vi "Programmablauf.vi"(8 "error in (no error)":errorcluster caption="Fehler (Eingang, kein Fehler)", 11 "AK Trigger":bool) -> (0 "error out":errorcluster caption="Fehler (Ausgang)")   [LabVIEW 2020, in "Schedule Modul.lvlib"]
uses:
  Schedule Modul.lvlib
  Aktion Trigger Freigabe.ctl
  Aktion FGV Testdaten sammeln.ctl
  T90/Aktion FGV Automatic Start.ctl
  Sprachverwaltung/FGV Aktion Tabelle zerlegen.ctl
  Aktion FGV Scheduler Status.ctl
  Aktion FGV Schedule Daten.ctl
  Funktionstasten/Funktionstasten-Aktion.ctl
  Funktionstasten/Zustaende.ctl
  Aktion FGV Schedule Log.ctl
  Auto Kalibrieren/VI Auto Kalibrieren.vi
  Seiten/Erweiterte Konfig/Dichtheitstest.vi
  Seiten/Erweiterte Konfig/Konfig CG-Check/CG-Test.vi
  T90/T90 main.vi
  Funktionstasten/Funktionstasten.lvlib
  Funktionstasten/Freigabe Aktionen.ctl
  AK-Schnittstelle/AK-Schnittstelle.lvlib
  Allgemein/allgemeine Sub-VIs.lvlib
  Seiten/Erweiterte Konfig/Erweiterte Konfig.lvlib
  Seiten/Erweiterte Konfig/Konfig CG-Check/CG-Check Konfig.lvlib
  T90/T90.lvlib
  Sprachverwaltung/Sprachverwaltung.lvlib
  Auto Kalibrieren/Auto Kalibrieren.lvlib
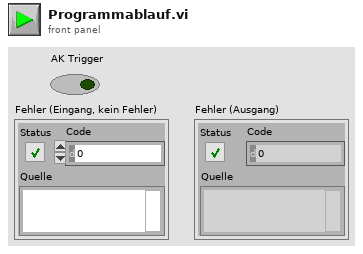
[diagram p1: front panel]
types:
  T1 = typedef "Schedule Modul.lvlib/Aktion FGV Scheduler Status.ctl" = enum16{"lesen", "init", "aktiv", "inaktiv"}
  T2 = typedef "Sprachverwaltung.lvlib/FGV Aktion Tabelle zerlegen.ctl" = enum16{"laden", "vereinzeln", "speichern"}
  T3 = typedef "T90.lvlib/Aktion FGV Automatic Start.ctl" = enum16{"lesen", "aktivieren", "deaktivieren"}
  T4 = typedef "Schedule Modul.lvlib/Aktion FGV Testdaten sammeln.ctl" = enum16{"lesen", "Dichtheitstest", "CalGasTest", "T90", "Kalibrieren", "init", "Kalender Daten"}
  T5 = typedef "Schedule Modul.lvlib/Aktion Trigger Freigabe.ctl" = enum16{"init", "lesen", "prüfen", "löschen"}
  T6 = typedef "Funktionstasten.lvlib/Freigabe Aktionen.ctl" = enum16{"prüfen", "Freigabe?", "lesen"}
  T7 = typedef "Schedule Modul.lvlib/Aktion FGV Schedule Daten.ctl" = enum16{"lesen", "laden", "speichern", "schreiben"}
  T8 = typedef "Schedule Modul.lvlib/Testreihenfolge.ctl" = cluster{"Test 1":T9, "Test 2":T9, "Test 3":T9, "Test 4":T9, "Test 5":T9}
  T9 = typedef "Schedule Modul.lvlib/Test-Auswahlfeld.ctl" = u16
  T10 = typedef "Funktionstasten.lvlib/Zustaende.ctl" = enum16{"Standby", "Pause", "Eco", "Messen", "Kalibrieren", "Spülen Filter", "Spülen Leitung", "Umgebungsluft", "0-Gas", "Cal-Gas", "CG zu PNS", "-------------", "Init 1", "Init 2", "Init 3", "Init 4", "Messen vorbereiten", "Messen durchführen", "Exit"}
  T11 = typedef "Funktionstasten.lvlib/Funktionstasten-Aktion.ctl" = enum16{"Initialisieren", "Zustand setzen", "Taste gedrückt", "Fehler speichern", "Lesen", "Manuell", "Remote", "Bitparallel", "Samplepoint", "Zeit Prüfen", "reset Umschalten"}
  T12 = typedef "Schedule Modul.lvlib/Aktion FGV Schedule Log.ctl" = enum16{"lesen", "neuer Eintrag", "laden", "löschen", "Anzeige löschen"}
  T13 = typedef "Schedule Modul.lvlib/Ergebnis Dichtheitstest.ctl" = cluster{"Druck FT-IR:":T14, "max. Anstieg:":T14, "Druckanstieg:":T14, "Zeitdauer:":T14, "Verstrichene Zeit:":T14, "Fehler":bool, "Unterdruck nicht erreicht ":bool}
  T14 = typedef "Zahlen-Ausgabefeld.ctl" = sgl
  T15 = typedef "Schedule Modul.lvlib/Ergebnis Kalibrieren.ctl" = cluster{"Fehler":bool, "CO2 H2O vergleich":bool}
  T16 = typedef "Schedule Modul.lvlib/Ergebnis CalGas Test.ctl" = cluster{"Istwerte":string[][], "Auswertung":string[][][], "Fehler":bool[], "Abweichung in %":string[][]}
  T17 = typedef "Schedule Modul.lvlib/Ergebnis T90.ctl" = cluster{"T90":waveform(sgl), "T10:":T14, "T50:":T14, "T90:":T14, "Rise Time":T14, "Leitungslänge":T18, "Fehler":bool}
  T18 = typedef "Zahlen-Eingabefeld.ctl" = sgl
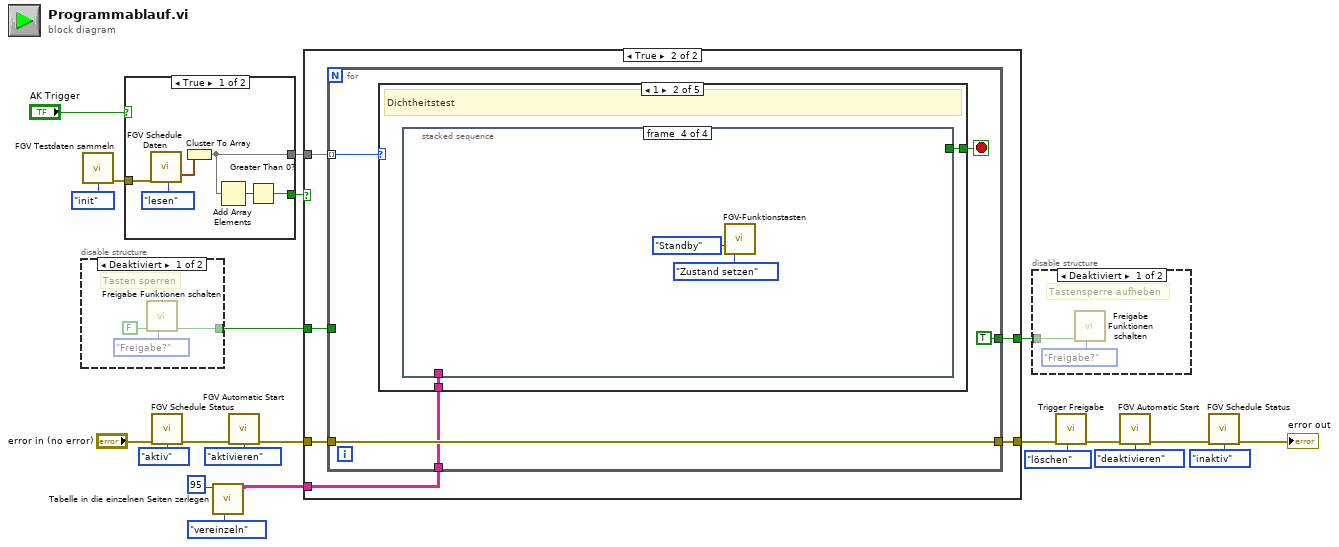
[diagram p0: block diagram]
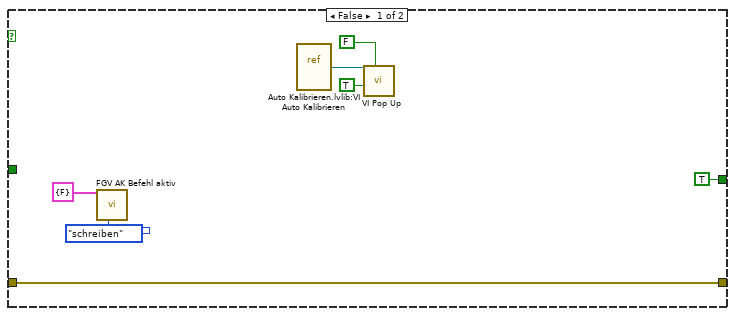
[diagram p4: hidden frame]
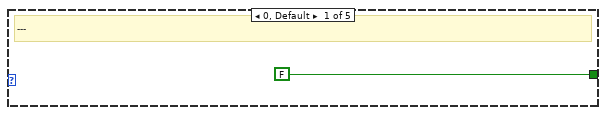
[diagram p5: hidden frame]
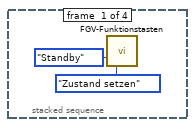
[diagram p6: hidden frame]
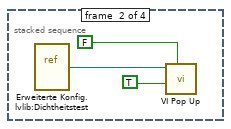
[diagram p7: hidden frame]
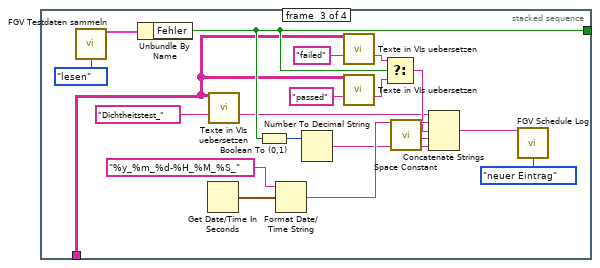
[diagram p8: hidden frame]
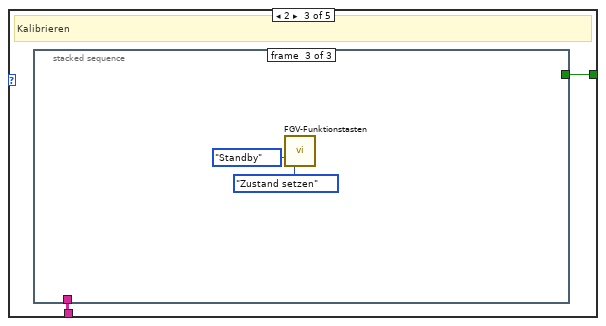
[diagram p9: hidden frame]
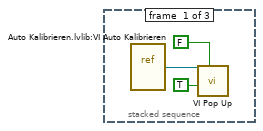
[diagram p10: hidden frame]
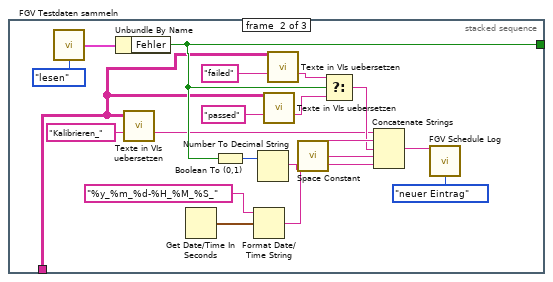
[diagram p11: hidden frame]
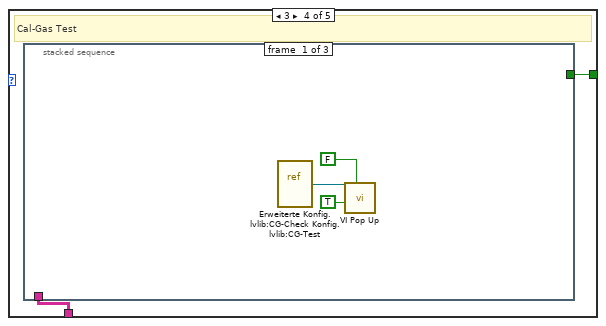
[diagram p12: hidden frame]
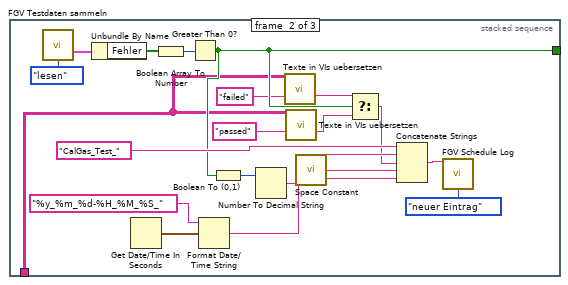
[diagram p13: hidden frame]
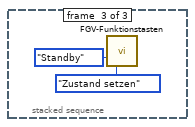
[diagram p14: hidden frame]
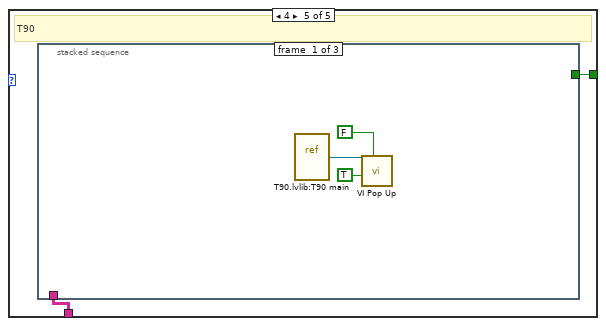
[diagram p15: hidden frame]
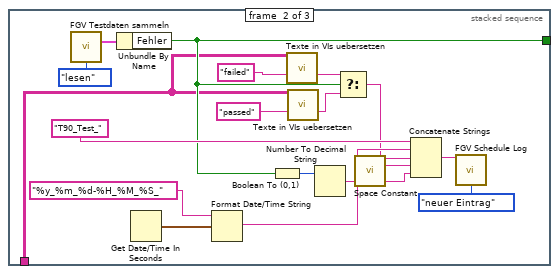
[diagram p16: hidden frame]
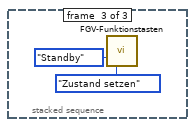
[diagram p17: hidden frame]
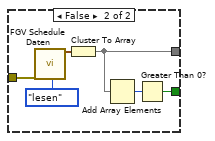
[diagram p18: hidden frame]
diagram:
  n1 = disable-structure shown="Deaktiviert" {
    disable-tunnel: [w25 _] -> w16
    frame Disabled {
      # "Tasten sperren"
      n2 = call "Freigabe Funktionen schalten.vi"("Aktionen"=Freigabe_Aktionen."Freigabe?", "Freigabe?"=FALSE) -> ("Freigabe?"=w25:bool)  [unwired: 7 in, 2 out]
    }
    frame Enabled {
    }
  }
  n3 = call "FGV Testdaten sammeln.vi"("Aktion"=Aktion_FGV_Testdaten_sammeln."init") -> ("error out"=w18:errorcluster)  [unwired: 9 in, 5 out]
  n4 = case shown="True" "AK Trigger" {
    tunnel: [w27 w32] -> w22
    tunnel: w18 -> [w30 w35]
    tunnel: [w26 w33] -> w14
    frame True {
      n5 = call "FGV Schedule Daten.vi"("error in (no error)"=w30, "Aktion"=Aktion_FGV_Schedule_Daten."lesen") -> ("Testreihenfolge AK"=w29:T8)  [unwired: 12 in, 5 out]
      n6 = Cluster To Array(cluster=w29) -> (array=w27:T9[])
      n7 = Add Array Elements(numeric array=w27) -> (sum=w28:T9)
      n8 = Greater Than 0?(x=w28) -> (x > 0?=w26:bool)
    }
    frame False {
      n9 = call "FGV Schedule Daten.vi"("error in (no error)"=w35, "Aktion"=Aktion_FGV_Schedule_Daten."lesen") -> ("Testreihenfolge:"=w36:T8)  [unwired: 12 in, 5 out]
      n10 = Cluster To Array(cluster=w36) -> (array=w32:T9[])
      n11 = Add Array Elements(numeric array=w32) -> (sum=w34:T9)
      n12 = Greater Than 0?(x=w34) -> (x > 0?=w33:bool)
    }
  }
  n13 = call "FGV Schedule Status.vi"("error in (no error)"="error in (no error)", "Aktion"=Aktion_FGV_Scheduler_Status."aktiv") -> ("error out"=w6:errorcluster)  [unwired: 12 in, 1 out]
  n14 = call "Tabelle in die einzelnen Seiten zerlegen.vi"("Aktion"=FGV_Aktion_Tabelle_zerlegen."vereinzeln", "Index (Seite)"=95) -> ("Sprachliste"=w7:string[][])  [unwired: 7 in, 2 out]
  n15 = call "FGV Automatic Start.vi"("error in (no error)"=w6, "Aktion"=Aktion_FGV_Automatic_Start."aktivieren") -> ("error out"=w13:errorcluster)  [unwired: 12 in, 1 out]
  n16 = case shown="True" w14 {
    tunnel: w22 -> [_ w50]
    tunnel: w13 -> [w43 w49]
    tunnel: [w43 w48] -> w20
    tunnel: w16 -> [_ w47]
    tunnel: [TRUE ("Freigabe?") w46] -> w15
    tunnel: w7 -> [_ w45]
    frame False {
      n17 = call "FGV AK Befehl aktiv.vi"("Aktion"=enum16{"initialisieren", "lesen", "schreiben"}."schreiben", "Cluster (in)"=cluster{"Befehl von AK":bool} {"Befehl von AK"=FALSE}) -> ()  [unwired: 9 in, 1 out]
      n18 = vi-ref "Auto Kalibrieren.lvlib:VI Auto Kalibrieren.vi"() -> (w40:refnum<vi>)
      n19 = call "VI Pop Up.vi"("Aufrufer gesperrt?"=FALSE, "Warten bis beendet"=TRUE, "VI Referenz"=w40) -> ()  [unwired: 9 in]
    }
    frame True {
      n20 = for {
        tunnel: w50 -> [w55] mode=indexing
        tunnel: w49 -> [w54]
        tunnel: [w54] -> w48
        tunnel: w47 -> [_]
        tunnel: [TRUE ("Freigabe?")] -> w46
        tunnel: w45 -> [w51]
        stop <- w53 stop-if-true
        n21 = case shown="1" w55 {
          tunnel: [FALSE ("Fehler") w58 w86 w112 w139] -> w53
          tunnel: w51 -> [_ w57 w85 w111 w138]
          frame 0, Default {
            # "---"
          }
          frame 1 {
            # "Dichtheitstest"
            n22 = stacked-sequence {
              tunnel: [_ _ w73 _] -> w58
              tunnel: w57 -> [_ _ w64 _]
              frame #0 {
                n23 = call "FGV-Funktionstasten.vi"("Zustand"=Zustaende."Standby", "Aktion"=Funktionstasten-Aktion."Zustand setzen") -> ()  [unwired: 6 in, 8 out]
              }
              frame #1 {
                n24 = vi-ref "Erweiterte Konfig.lvlib:Dichtheitstest.vi"() -> (w63:refnum<vi>)
                n25 = call "VI Pop Up.vi"("Aufrufer gesperrt?"=FALSE, "Warten bis beendet"=TRUE, "VI Referenz"=w63) -> ()  [unwired: 9 in]
              }
              frame #2 {
                n26 = call "FGV Testdaten sammeln.vi"("Aktion"=Aktion_FGV_Testdaten_sammeln."lesen") -> ("Ergebnisse Dichtheitstest"=w81:T13)  [unwired: 9 in, 5 out]
                n27 = Unbundle By Name(w81) -> ("Fehler"=w73:bool)
                n28 = Get Date/Time In Seconds() -> (seconds since 1Jan1904=w79:timestamp)
                n29 = call "Texte in VIs uebersetzen.vi"("Sprachliste"=w64, "String zum Übersetzen"="Dichtheitstest_") -> ("String zum Übersetzen"=w69:string)  [unwired: 9 in, 4 out]
                n30 = Boolean To (0,1)(Boolean=w73) -> (0, 1=w76:i16)
                n31 = Format Date/Time String(time format string (%c)="%y_%m_%d-%H_%M_%S_" ("Zeitformatierungs-String (%c)"), seconds (now)=w79) -> (date/time string=w78:string)  [unwired: 1 in]
                n32 = Number To Decimal String(number=w76) -> (decimal integer string=w74:string)  [unwired: 1 in]
                n33 = call "Texte in VIs uebersetzen.vi"("Sprachliste"=w64, "String zum Übersetzen"="failed") -> ("String zum Übersetzen"=w68:string)  [unwired: 9 in, 4 out]
                n34 = call "Texte in VIs uebersetzen.vi"("Sprachliste"=w64, "String zum Übersetzen"="passed") -> ("String zum Übersetzen"=w66:string)  [unwired: 9 in, 4 out]
                n35 = Select(t=w68, s=w73, f=w66) -> (s? t:f=w77:string)
                n36 = call <vilib>:"Space Constant.vi"() -> ("String"=w75:string)
                n37 = Concatenate Strings(w69, w78, w77, w75, w74) -> (w71:string)
                n38 = call "FGV Schedule Log.vi"("Neuer Eintrag"=w71, "Aktion"=Aktion_FGV_Schedule_Log."neuer Eintrag") -> ()  [unwired: 10 in, 4 out]
              }
              frame #3 {
                n39 = call "FGV-Funktionstasten.vi"("Zustand"=Zustaende."Standby", "Aktion"=Funktionstasten-Aktion."Zustand setzen") -> ()  [unwired: 6 in, 8 out]
              }
            }
          }
          frame 2 {
            # "Kalibrieren"
            n40 = stacked-sequence {
              tunnel: [_ w99 _] -> w86
              tunnel: w85 -> [_ w90 _]
              frame #0 {
                n41 = vi-ref "Auto Kalibrieren.lvlib:VI Auto Kalibrieren.vi"() -> (w89:refnum<vi>)
                n42 = call "VI Pop Up.vi"("Aufrufer gesperrt?"=FALSE, "Warten bis beendet"=TRUE, "VI Referenz"=w89) -> ()  [unwired: 9 in]
              }
              frame #1 {
                n43 = call "FGV Testdaten sammeln.vi"("Aktion"=Aktion_FGV_Testdaten_sammeln."lesen") -> ("Ergebnisse Kalibrieren"=w107:T15)  [unwired: 9 in, 5 out]
                n44 = Unbundle By Name(w107) -> ("Fehler"=w99:bool)
                n45 = call "Texte in VIs uebersetzen.vi"("Sprachliste"=w90, "String zum Übersetzen"="Kalibrieren_") -> ("String zum Übersetzen"=w95:string)  [unwired: 9 in, 4 out]
                n46 = Get Date/Time In Seconds() -> (seconds since 1Jan1904=w105:timestamp)
                n47 = Boolean To (0,1)(Boolean=w99) -> (0, 1=w102:i16)
                n48 = Format Date/Time String(time format string (%c)="%y_%m_%d-%H_%M_%S_" ("Zeitformatierungs-String (%c)"), seconds (now)=w105) -> (date/time string=w104:string)  [unwired: 1 in]
                n49 = Number To Decimal String(number=w102) -> (decimal integer string=w100:string)  [unwired: 1 in]
                n50 = call "Texte in VIs uebersetzen.vi"("Sprachliste"=w90, "String zum Übersetzen"="passed") -> ("String zum Übersetzen"=w92:string)  [unwired: 9 in, 4 out]
                n51 = call "Texte in VIs uebersetzen.vi"("Sprachliste"=w90, "String zum Übersetzen"="failed") -> ("String zum Übersetzen"=w91:string)  [unwired: 9 in, 4 out]
                n52 = call <vilib>:"Space Constant.vi"() -> ("String"=w101:string)
                n53 = Select(t=w91, s=w99, f=w92) -> (s? t:f=w103:string)
                n54 = Concatenate Strings(w95, w104, w103, w101, w100) -> (w97:string)
                n55 = call "FGV Schedule Log.vi"("Neuer Eintrag"=w97, "Aktion"=Aktion_FGV_Schedule_Log."neuer Eintrag") -> ()  [unwired: 10 in, 4 out]
              }
              frame #2 {
                n56 = call "FGV-Funktionstasten.vi"("Zustand"=Zustaende."Standby", "Aktion"=Funktionstasten-Aktion."Zustand setzen") -> ()  [unwired: 6 in, 8 out]
              }
            }
          }
          frame 3 {
            # "Cal-Gas Test"
            n57 = stacked-sequence {
              tunnel: [_ w124 _] -> w112
              tunnel: w111 -> [_ w116 _]
              frame #0 {
                n58 = vi-ref "Erweiterte Konfig.lvlib:CG-Check Konfig.lvlib:CG-Test.vi"() -> (w115:refnum<vi>)
                n59 = call "VI Pop Up.vi"("Aufrufer gesperrt?"=FALSE, "Warten bis beendet"=TRUE, "VI Referenz"=w115) -> ()  [unwired: 9 in]
              }
              frame #1 {
                n60 = call "FGV Testdaten sammeln.vi"("Aktion"=Aktion_FGV_Testdaten_sammeln."lesen") -> ("Ergebnis CalGas Test"=w135:T16)  [unwired: 9 in, 5 out]
                n61 = Unbundle By Name(w135) -> ("Fehler"=w133:bool[])
                n62 = Get Date/Time In Seconds() -> (seconds since 1Jan1904=w130:timestamp)
                n63 = Boolean Array To Number(Boolean array=w133) -> (number=w132:u32)
                n64 = Greater Than 0?(x=w132) -> (x > 0?=w124:bool)
                n65 = Format Date/Time String(time format string (%c)="%y_%m_%d-%H_%M_%S_" ("Zeitformatierungs-String (%c)"), seconds (now)=w130) -> (date/time string=w128:string)  [unwired: 1 in]
                n66 = Boolean To (0,1)(Boolean=w124) -> (0, 1=w126:i16)
                n67 = Number To Decimal String(number=w126) -> (decimal integer string=w123:string)  [unwired: 1 in]
                n68 = call "Texte in VIs uebersetzen.vi"("Sprachliste"=w116, "String zum Übersetzen"="failed") -> ("String zum Übersetzen"=w119:string)  [unwired: 9 in, 4 out]
                n69 = call "Texte in VIs uebersetzen.vi"("Sprachliste"=w116, "String zum Übersetzen"="passed") -> ("String zum Übersetzen"=w117:string)  [unwired: 9 in, 4 out]
                n70 = call <vilib>:"Space Constant.vi"() -> ("String"=w125:string)
                n71 = Select(t=w119, s=w124, f=w117) -> (s? t:f=w127:string)
                n72 = Concatenate Strings("CalGas_Test_", w128, w127, w125, w123) -> (w121:string)
                n73 = call "FGV Schedule Log.vi"("Neuer Eintrag"=w121, "Aktion"=Aktion_FGV_Schedule_Log."neuer Eintrag") -> ()  [unwired: 10 in, 4 out]
              }
              frame #2 {
                n74 = call "FGV-Funktionstasten.vi"("Zustand"=Zustaende."Standby", "Aktion"=Funktionstasten-Aktion."Zustand setzen") -> ()  [unwired: 6 in, 8 out]
              }
            }
          }
          frame 4 {
            # "T90"
            n75 = stacked-sequence {
              tunnel: [_ w152 _] -> w139
              tunnel: w138 -> [_ w143 _]
              frame #0 {
                n76 = vi-ref "T90.lvlib:T90 main.vi"() -> (w142:refnum<vi>)
                n77 = call "VI Pop Up.vi"("Aufrufer gesperrt?"=FALSE, "Warten bis beendet"=TRUE, "VI Referenz"=w142) -> ()  [unwired: 9 in]
              }
              frame #1 {
                n78 = call "FGV Testdaten sammeln.vi"("Aktion"=Aktion_FGV_Testdaten_sammeln."lesen") -> ("Ergebnis T90"=w160:T17)  [unwired: 9 in, 5 out]
                n79 = Unbundle By Name(w160) -> ("Fehler"=w152:bool)
                n80 = Get Date/Time In Seconds() -> (seconds since 1Jan1904=w157:timestamp)
                n81 = Format Date/Time String(time format string (%c)="%y_%m_%d-%H_%M_%S_" ("Zeitformatierungs-String (%c)"), seconds (now)=w157) -> (date/time string=w155:string)  [unwired: 1 in]
                n82 = Boolean To (0,1)(Boolean=w152) -> (0, 1=w151:i16)
                n83 = call "Texte in VIs uebersetzen.vi"("Sprachliste"=w143, "String zum Übersetzen"="failed") -> ("String zum Übersetzen"=w145:string)  [unwired: 9 in, 4 out]
                n84 = call "Texte in VIs uebersetzen.vi"("Sprachliste"=w143, "String zum Übersetzen"="passed") -> ("String zum Übersetzen"=w144:string)  [unwired: 9 in, 4 out]
                n85 = Number To Decimal String(number=w151) -> (decimal integer string=w150:string)  [unwired: 1 in]
                n86 = Select(t=w145, s=w152, f=w144) -> (s? t:f=w154:string)
                n87 = call <vilib>:"Space Constant.vi"() -> ("String"=w153:string)
                n88 = Concatenate Strings("T90_Test_", w155, w154, w153, w150) -> (w148:string)
                n89 = call "FGV Schedule Log.vi"("Neuer Eintrag"=w148, "Aktion"=Aktion_FGV_Schedule_Log."neuer Eintrag") -> ()  [unwired: 10 in, 4 out]
              }
              frame #2 {
                n90 = call "FGV-Funktionstasten.vi"("Zustand"=Zustaende."Standby", "Aktion"=Funktionstasten-Aktion."Zustand setzen") -> ()  [unwired: 6 in, 8 out]
              }
            }
          }
        }
      }
    }
  }
  n91 = disable-structure shown="Deaktiviert" {
    disable-tunnel: w15 -> [w164 _]
    frame Disabled {
      # "Tastensperre aufheben"
      n92 = call "Freigabe Funktionen schalten.vi"("Aktionen"=Freigabe_Aktionen."Freigabe?", "Freigabe?"=w164) -> ()  [unwired: 7 in, 3 out]
    }
    frame Enabled {
    }
  }
  n93 = call "Trigger Freigabe.vi"("Aktion"=Aktion_Trigger_Freigabe."löschen", "error in (no error)"=w20) -> ("error out"=w12:errorcluster)  [unwired: 8 in, 1 out]
  n94 = call "FGV Automatic Start.vi"("error in (no error)"=w12, "Aktion"=Aktion_FGV_Automatic_Start."deaktivieren") -> ("error out"=w3:errorcluster)  [unwired: 12 in, 1 out]
  n95 = call "FGV Schedule Status.vi"("error in (no error)"=w3, "Aktion"=Aktion_FGV_Scheduler_Status."inaktiv") -> ("error out"=→"error out":errorcluster)  [unwired: 12 in, 1 out]
